vi "SDSU_Reg_Value2Fields.vi"(8 "error in (no error)":errorcluster, 9 "value":i32, 10 "Register":T1) -> (0 "error out":errorcluster, 2 "Register out":T1)   [LabVIEW 2016]
uses:
  SDSU_Register.ctl
  SDSU_RegField.ctl
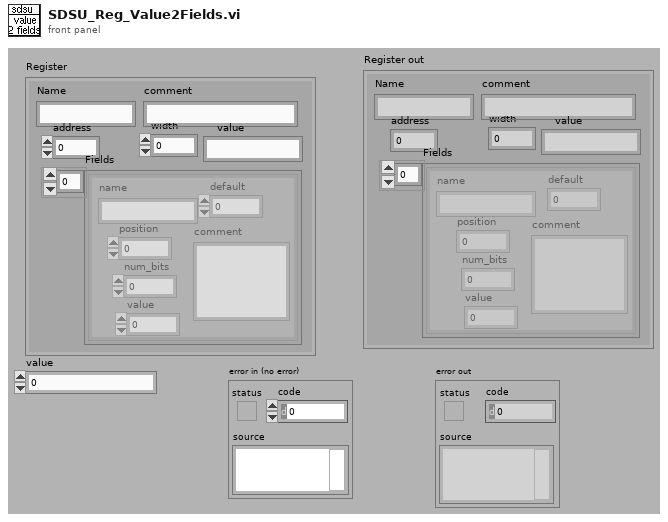
[diagram p1: front panel]
types:
  T1 = typedef "SDSU_Register.ctl" = cluster{"Name":string, "address":i16, "width":i16, "comment":string, "Fields":T2[], "value":string}
  T2 = typedef "SDSU_RegField.ctl" = cluster{"name":string, "position":u16, "num_bits":u16, "default":i16, "comment":string, "value":i32}
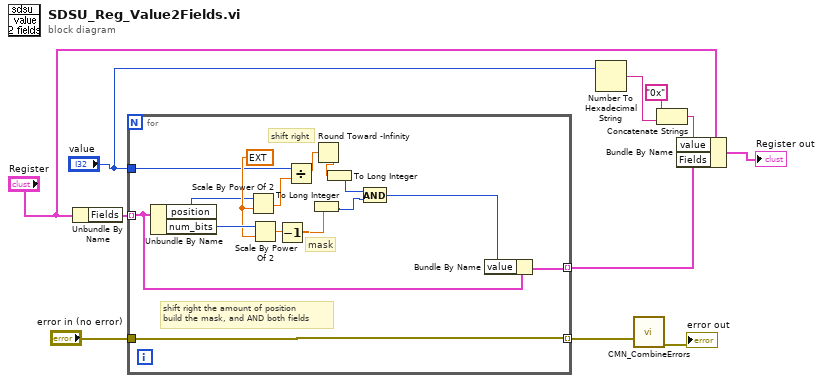
[diagram p0: block diagram]
diagram:
  n1 = Unbundle By Name("Register") -> ("Fields"=w11:T2[])
  n2 = for {
    tunnel: w11 -> [w16] mode=indexing
    tunnel: "error in (no error)" -> [w22]
    tunnel: [w22] -> w7 mode=indexing
    tunnel: "value" -> [w18]
    tunnel: [w15] -> w5 mode=indexing
    w24 = ext 1.0 ("x")
    # "shift right the amount of position\nbuild the mask, and AND both fields"
    # "mask"
    # "shift right"
    n3 = Unbundle By Name(w16) -> ("position"=w23:u16, "num_bits"=w26:u16)
    n4 = Scale By Power Of 2(n=w23, x=w24) -> (x*2^n=w20:ext)
    n5 = Scale By Power Of 2(n=w26, x=w24) -> (x*2^n=w25:ext)
    n6 = Decrement(x=w25) -> (x-1=w21:ext)
    n7 = Divide(x=w18, y=w20) -> (x/y=w13:ext)
    n8 = To Long Integer(number=w21) -> (32bit integer=w17:i32)
    n9 = Round Toward -Infinity(1:w13) -> (0:w12:ext)
    n10 = To Long Integer(number=w12) -> (32bit integer=w19:i32)
    n11 = And(x=w19, y=w17) -> (x .and. y?=w14:i32)
    n12 = Bundle By Name(cluster=w16, "value"=w14) -> (w15:T2)
  }
  n13 = Number To Hexadecimal String(2:"value") -> (0:w2:string)  [unwired: 1 out]
  n14 = call "CMN_CombineErrors.vi"("Errors"=w7) -> ("error out"=→"error out":errorcluster)  [unwired: 10 out]
  n15 = Concatenate Strings("0x" ("string"), w2) -> (w1:string)
  n16 = Bundle By Name(cluster="Register", "value"=w1, "Fields"=w5) -> (→"Register out":T1)
